vi "Dependency Create Parameters.vi"(5 "Common Doc Dir":string, 7 "CD Name":string, 10 "Generated Files in":string[](array[string])) -> (2 "Dependency Parameters":T1[](array[typedef]))   [LabVIEW 2018, in ".LVLIBP CD XML Updater.lvlib" / "Project XML Editor.lvclass"]
uses:
  Project XML Editor.lvclass
  TypeDefs/Dependency Parameters.ctl
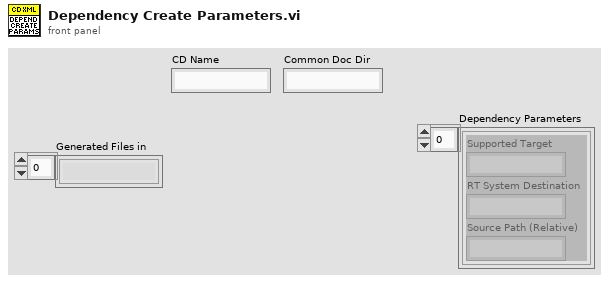
[diagram p1: front panel]
types:
  T1 = typedef ".LVLIBP CD XML Updater.lvlib/Project XML Editor.lvclass/Dependency Parameters.ctl" = cluster{"Supported Target":string, "RT System Destination":string, "Source Path (Relative)":string}
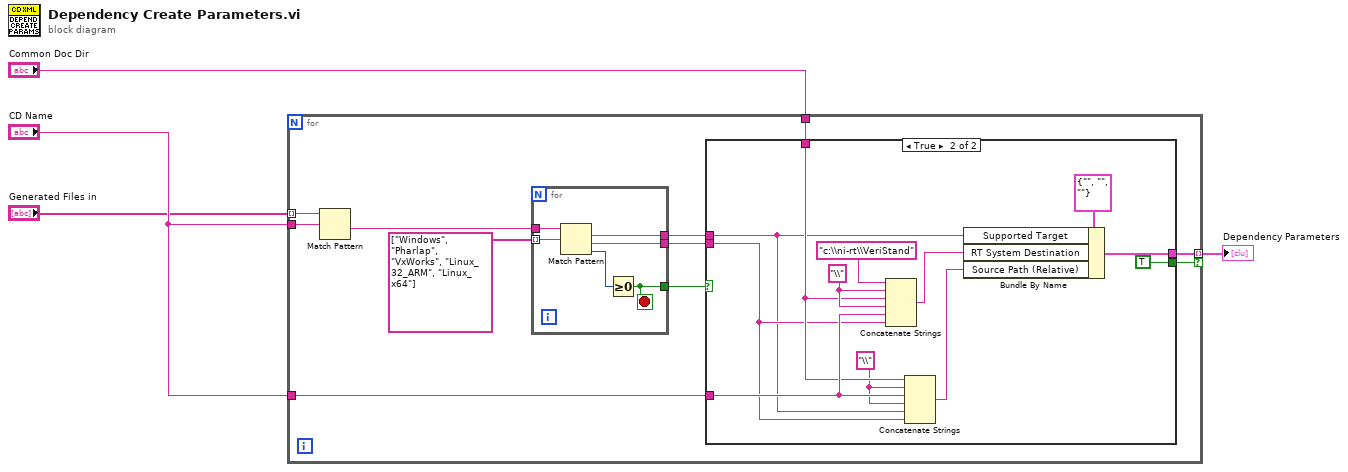
[diagram p0: block diagram]
diagram:
  n1 = for {
    tunnel: "Generated Files in" -> [w15] mode=indexing
    tunnel: "CD Name" -> [w14]
    tunnel: "CD Name" -> [w10]
    tunnel: [w11] -> w2 mode=indexing if=w5
    tunnel: "Common Doc Dir" -> [w9]
    n2 = Match Pattern(string=w15, regular expression=w14) -> (after substring=w13:string)  [unwired: 1 in, 3 out]
    n3 = for {
      tunnel: w13 -> [w33]
      tunnel: string[] ["Windows", "Pharlap", "VxWorks", "Linux_32_ARM", "Linux_x64"] -> [w32] mode=indexing
      tunnel: [w30] -> w7
      tunnel: [w29] -> w8
      tunnel: [w28] -> w6
      stop <- w28 stop-if-true
      n4 = Match Pattern(string=w33, regular expression=w32) -> (match substring=w30:string, after substring=w29:string, offset past match=w31:i32)  [unwired: 1 in, 1 out]
      n5 = Greater Or Equal To 0?(x=w31) -> (x >= 0?=w28:bool)
    }
    n6 = case shown="True" w6 {
      tunnel: [_ w24] -> w11
      tunnel: w10 -> [_ w21]
      tunnel: w9 -> [_ w20]
      tunnel: w8 -> [_ w18]
      tunnel: w7 -> [_ w17]
      tunnel: [_ TRUE] -> w5
      frame False {
      }
      frame True {
        w22 = "\\" ("string")
        w19 = "\\" ("string")
        n7 = Concatenate Strings("c:\\ni-rt\\VeriStand" ("string"), w22, w20, w22, w21, w18) -> (w26:string)
        n8 = Concatenate Strings(w20, w19, w21, w19, w17, w18) -> (w25:string)
        n9 = Bundle By Name(cluster=T1 {"Supported Target"="", "RT System Destination"="", "Source Path (Relative)"=""} ("Dependency Parameters"), "Supported Target"=w17, "RT System Destination"=w26, "Source Path (Relative)"=w25) -> (w24:T1)
      }
    }
  }
  "Dependency Parameters" <- w2
